vi "_RT_CtrlLoop_Log setLogMessage.vi"(7 "system type":T1, 8 "error in":errorcluster, 10 "customErrorMsg":string, 11 "RTLogQueue in":refnum<queue>) -> (0 "error out":errorcluster, 3 "RTLogQueue out":refnum<queue>)   [LabVIEW 2018]
uses:
  PublicSubVI/Ctl/_ctl_RT_SysLog.ctl
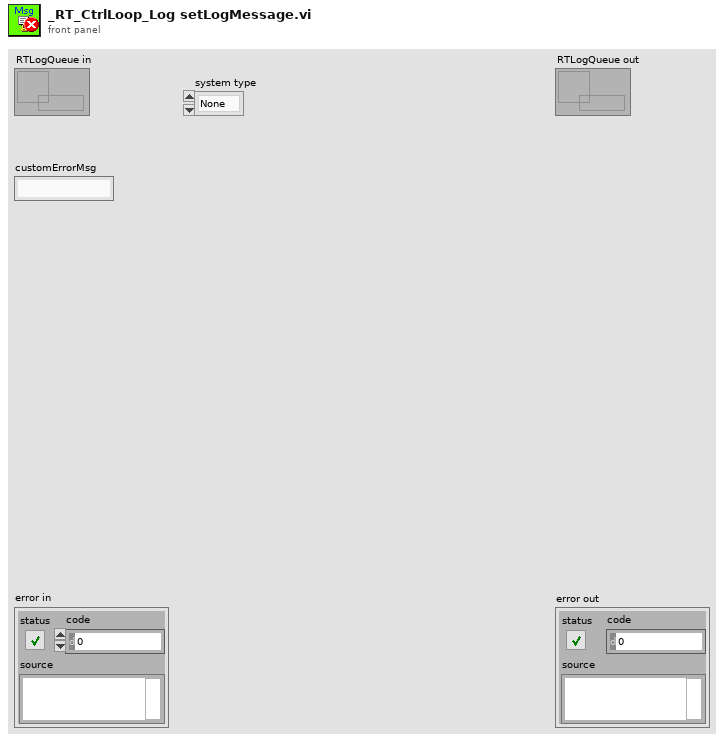
[diagram p1: front panel]
types:
  T1 = typedef "_ctl_RT_SysLog.ctl" = enum16{"None", "Initialize", "StartupRT", "StartupFPGA", "StartupAllocator", "GetMass", "SetWfmCode", "SetLaserCtrl", "SetTurboCtrl", "SetD999Ctrl", "Reconnecting...", "Interrupt", "StopRT"}
  T2 = cluster{"function type":enum16{"none", "init", "write", "read"}, "actionCmd":string, "callChain":string, "customErrorMsg":string, "error constant":errorcluster}
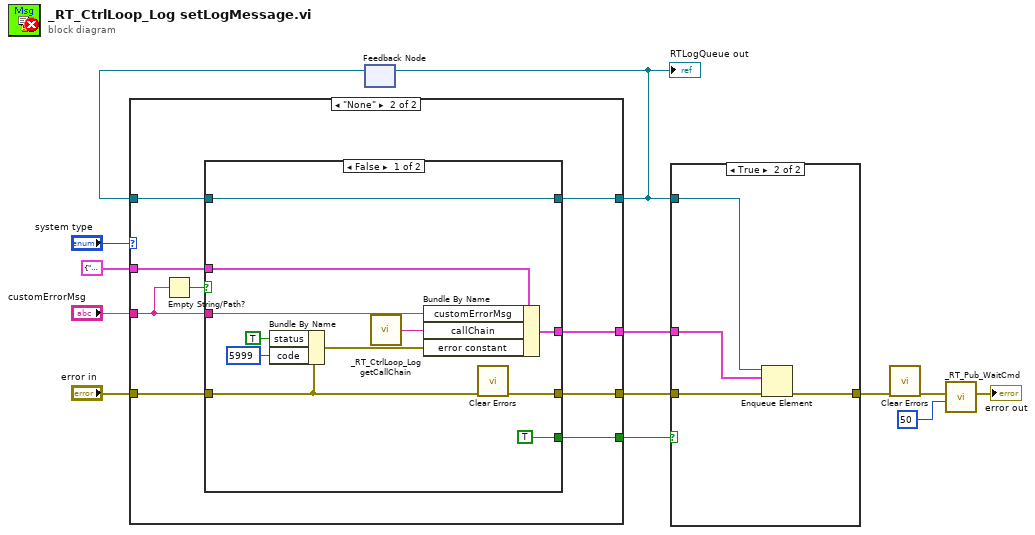
[diagram p0: block diagram]
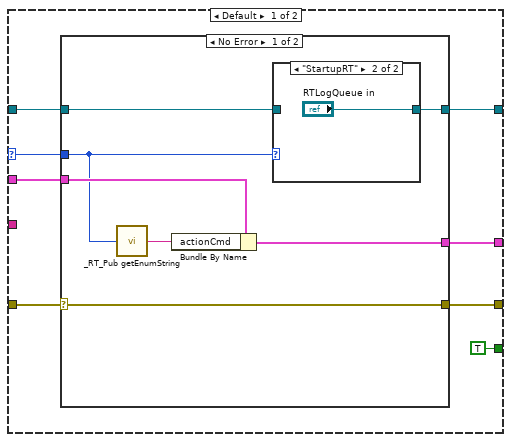
[diagram p3: hidden frame]
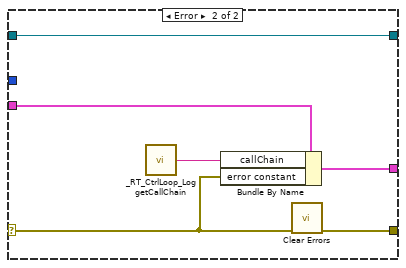
[diagram p5: hidden frame]
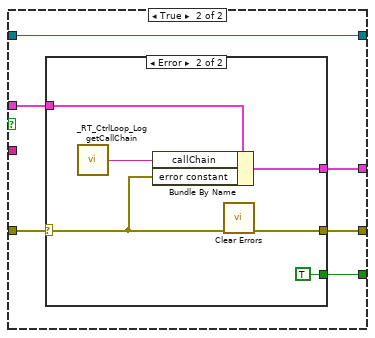
[diagram p6: hidden frame]
diagram:
  n1 = feedback #1() -> (w7:refnum<queue>)  [unwired: 1 in]
  n2 = case shown="\"None\"" "system type" {
    selector: "system type" -> [w21 _]
    tunnel: "error in" -> [w18 w41]
    tunnel: T2 {"function type"=enum."write", "actionCmd"="", "callChain"="", "customErrorMsg"="", "error constant"={"status"=FALSE, "code"=0, "source"=""}} ("element") -> [w20 w43]
    tunnel: [w17 w40] -> w4
    tunnel: [w19 w42] -> w5
    tunnel: "customErrorMsg" -> [_ w44]
    tunnel: [TRUE w39] -> w6
    tunnel: [w15 w38] -> w1
    tunnel: w7 -> [w14 w37]
    frame Default {
      n3 = case shown="No Error" w18 {
        selector: w18 -> [w25 w34]
        tunnel: w21 -> [w24 _]
        tunnel: w20 -> [w28 w35]
        tunnel: [w26 w32] -> w19
        tunnel: [w25 w33] -> w17
        tunnel: [w23 w31] -> w15
        tunnel: w14 -> [w22 w31]
        frame No Error {
          n4 = call "_RT_Pub getEnumString.vi"("system type"=w24) -> ("element"=w27:string)
          n5 = Bundle By Name(cluster=w28, "actionCmd"=w27) -> (w26:T2)
          n6 = case shown="\"StartupRT\"" w24 {
            tunnel: [w29 "RTLogQueue in"] -> w23
            tunnel: w22 -> [w29 _]
            frame Default {
            }
            frame "StartupRT" {
            }
          }
        }
        frame Error {
          n7 = call "_RT_CtrlLoop_Log getCallChain.vi"() -> ("callChainString"=w36:string)
          n8 = Bundle By Name(cluster=w35, "callChain"=w36, "error constant"=w34) -> (w32:T2)
          n9 = call <vilib>:"Clear Errors.vi"("error in (no error)"=w34) -> ("error out"=w33:errorcluster)  [unwired: 5 in, 1 out]
        }
      }
    }
    frame "None" {
      n10 = Empty String/Path?(string/path=w44) -> (empty?=w45:bool)
      n11 = case shown="False" w45 {
        tunnel: w44 -> [w55 _]
        tunnel: w43 -> [w56 w61]
        tunnel: [w54 w59] -> w42
        tunnel: w41 -> [w49 w62]
        tunnel: [w48 w60] -> w40
        tunnel: [TRUE w58] -> w39
        tunnel: [w46 w57] -> w38
        tunnel: w37 -> [w46 w57]
        frame False {
          n12 = Bundle By Name(cluster=w49, "status"=TRUE, "code"=5999) -> (w50:errorcluster)
          n13 = call "_RT_CtrlLoop_Log getCallChain.vi"() -> ("callChainString"=w53:string)
          n14 = Bundle By Name(cluster=w56, "customErrorMsg"=w55, "callChain"=w53, "error constant"=w50) -> (w54:T2)
          n15 = call <vilib>:"Clear Errors.vi"("error in (no error)"=w49) -> ("error out"=w48:errorcluster)  [unwired: 5 in, 1 out]
        }
        frame True {
          n16 = case shown="Error" w62 {
            selector: w62 -> [w63 w67]
            tunnel: w61 -> [_ w69]
            tunnel: [w63 w66] -> w60
            tunnel: [_ w65] -> w59
            tunnel: [_ TRUE] -> w58
            frame No Error {
            }
            frame Error {
              n17 = call "_RT_CtrlLoop_Log getCallChain.vi"() -> ("callChainString"=w68:string)
              n18 = Bundle By Name(cluster=w69, "callChain"=w68, "error constant"=w67) -> (w65:T2)
              n19 = call <vilib>:"Clear Errors.vi"("error in (no error)"=w67) -> ("error out"=w66:errorcluster)  [unwired: 5 in, 1 out]
            }
          }
        }
      }
    }
  }
  "RTLogQueue out" <- w1
  n20 = feedback-in #1(w1) -> ()
  n21 = case shown="True" w6 {
    tunnel: w1 -> [_ w73]
    tunnel: w5 -> [_ w72]
    tunnel: w4 -> [w70 w74]
    tunnel: [w70 w71] -> w3
    frame False {
    }
    frame True {
      n22 = Enqueue Element(queue=w73, element=w72, error in (no error)=w74) -> (error out=w71:errorcluster)  [unwired: 1 in, 2 out]
    }
  }
  n23 = call <vilib>:"Clear Errors.vi"("error in (no error)"=w3) -> ("error out"=w2:errorcluster)  [unwired: 5 in, 1 out]
  n24 = call "_RT_Pub_WaitCmd.vi"("milliseconds to wait"=u32 50, "error in (no error)"=w2) -> ("error out"=→"error out":errorcluster)  [unwired: 9 in]
